vi "TRACEABILITY.vi"() -> ()   [LabVIEW 2017]
uses:
  <vilib>/addons/database/Connection.llb/DB Tools Open Connec (String).vi
  Global/Global 1.vi
  <vilib>/addons/database/NI_Database_API.lvlib
panel:
  in  "Cluster":T1
  out "error out":errorcluster
  in  "error in (no error)":errorcluster
  in  "SAVE":bool
  in  "EXIT":bool
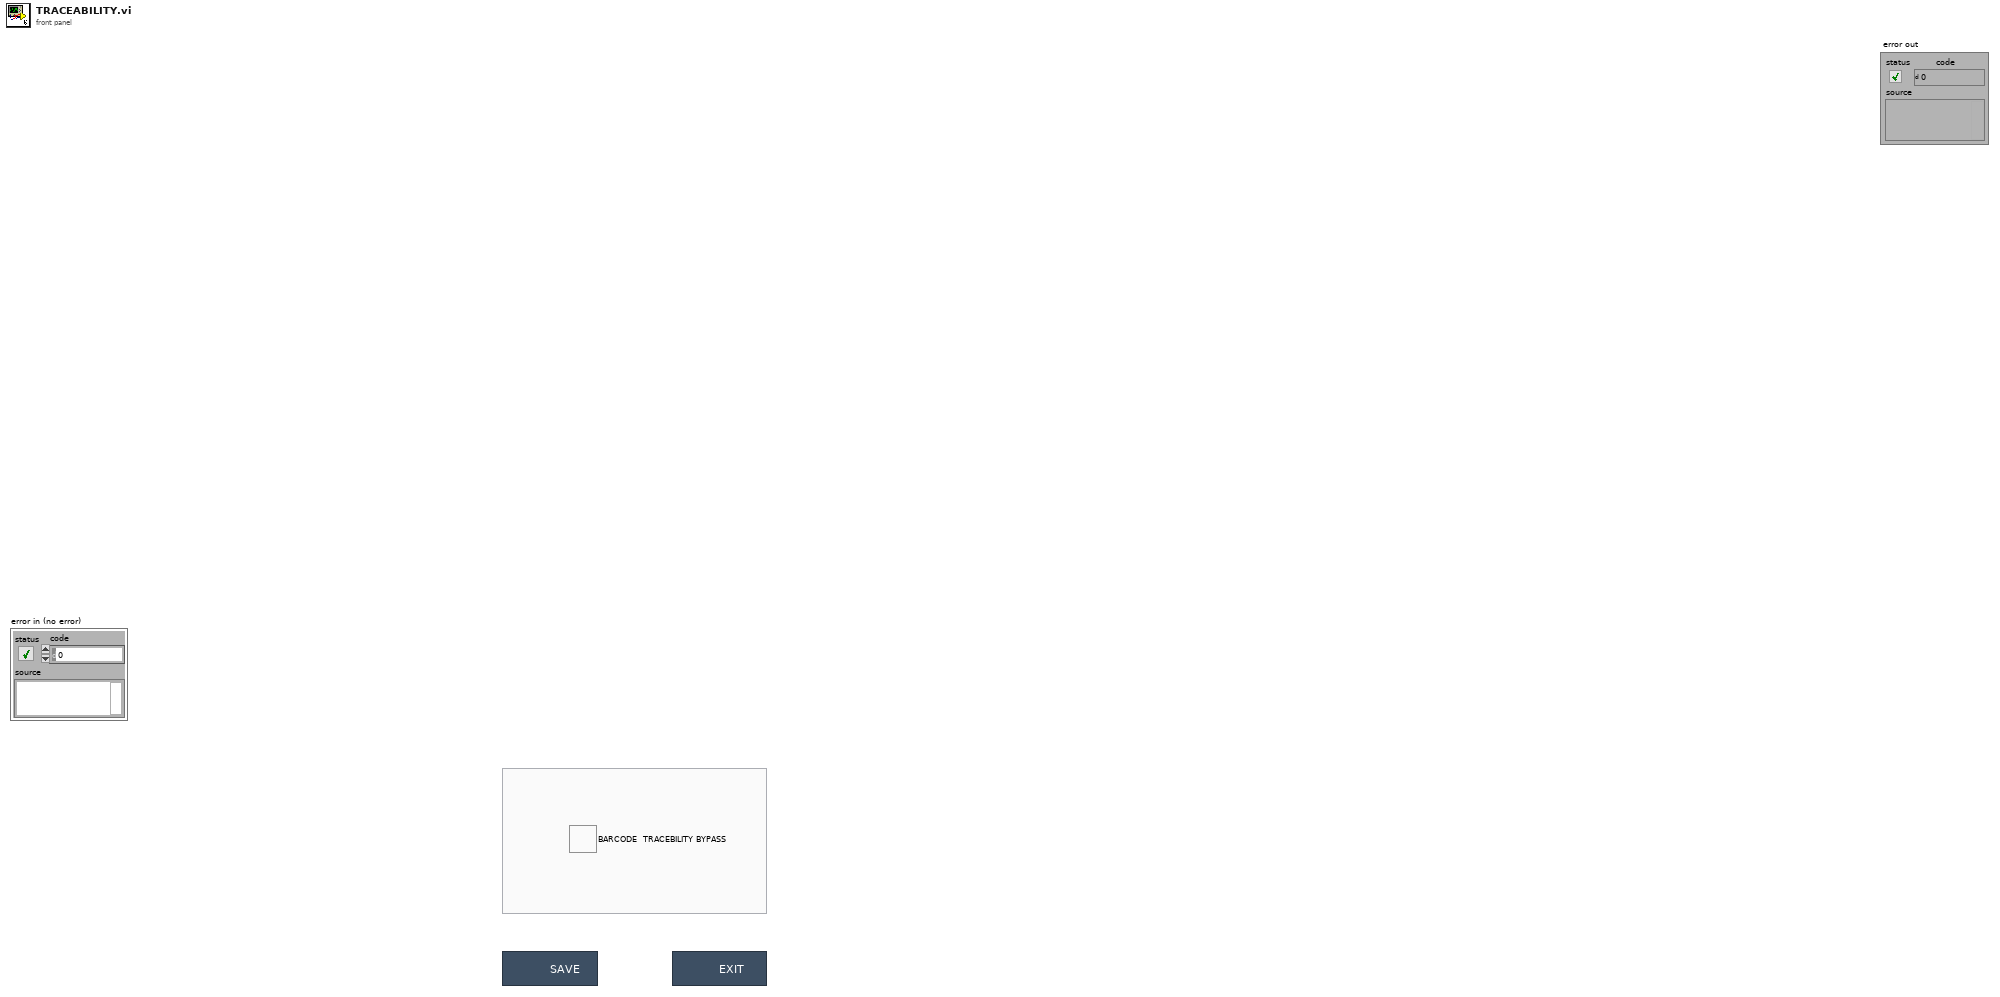
[diagram p1: front panel]
types:
  T1 = cluster{"BARCODE  TRACEBILITY BYPASS":bool, "BOM TRACEABILITY ":bool}
  T2 = cluster{"BARCODE TRACEABILITY":bool, "BOM TRACEABILITY ":bool}
  T3 = typedef "NI_Database_API.lvlib/Conn ObjectReference.ctl" = refnum<k1>
  T4 = enum32{"invalid app kind", "Development System", "Run Time System", "Student Edition", "Embedded LabVIEW", "Evaluation", "Custom"}
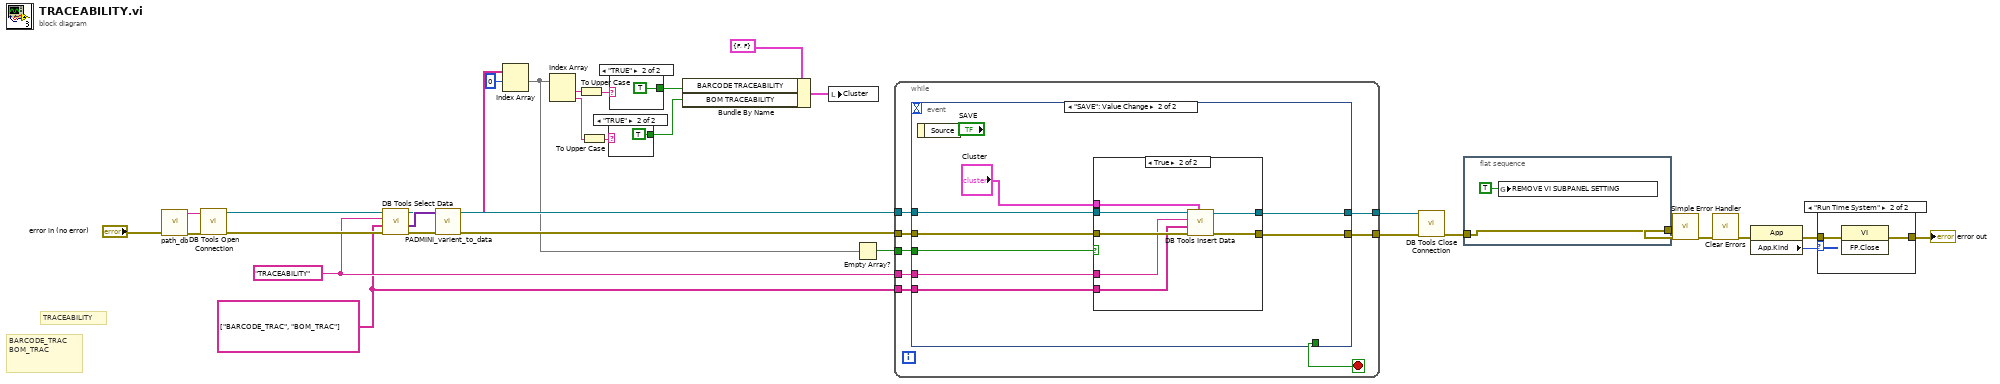
[diagram p0: block diagram]
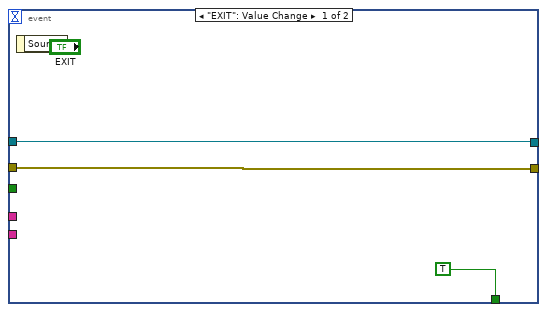
[diagram p2: hidden frame]
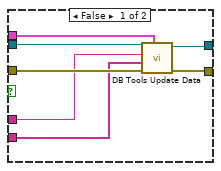
[diagram p3: hidden frame]
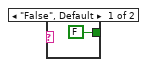
[diagram p5: hidden frame]
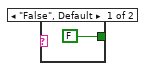
[diagram p6: hidden frame]
diagram:
  w12 = string[] ["BARCODE_TRAC", "BOM_TRAC"] ("columns")
  w13 = "TRACEABILITY" ("table")
  # "BARCODE_TRAC\nBOM_TRAC"
  # "TRACEABILITY"
  n1 = call "path_db.vi"("error in"="error in (no error)") -> ("error out"=w19:errorcluster, "resulting string"=w24:string)  [unwired: 9 in]
  n2 = call-poly <vilib>:"DB Tools Open Connection.vi"("error in (no error)"=w19, "connection information"=w24) -> ("error out"=w23:errorcluster, "connection reference"=w22:T3)  [unwired: 6 in]
  n3 = call <vilib>:"DB Tools Select Data.vi"("error in (no error)"=w23, "columns"=w12, "table"=w13, "connection reference"=w22) -> ("error out"=w21:errorcluster, "data"=w20:variant[][], "connection reference out"=w17:T3)  [unwired: 2 in]
  n4 = call "PADMINI_varient_to_data.vi"("error in (no error)"=w21, "data"=w20) -> ("error out"=w18:errorcluster, "Array"=w15:string[][])  [unwired: 8 in]
  n5 = Index Array(array=w15, index (row)=0 ("disabled index (col)")) -> (element=w14:string[])  [unwired: 1 in]
  n6 = Index Array(array=w14) -> (element #1=w6:string, element #2=w4:string)  [unwired: 2 in]
  n7 = To Upper Case(1:w6) -> (0:w2:string)
  n8 = To Upper Case(1:w4) -> (0:w1:string)
  n9 = case shown="\"TRUE\"" w1 {
    tunnel: [FALSE ("BARCODE TRACEABILITY") TRUE ("BARCODE TRACEABILITY")] -> w3
    frame "False", Default {
    }
    frame "TRUE" {
    }
  }
  n10 = case shown="\"TRUE\"" w2 {
    tunnel: [FALSE ("BARCODE TRACEABILITY") TRUE ("BARCODE TRACEABILITY")] -> w5
    frame "False", Default {
    }
    frame "TRUE" {
    }
  }
  n11 = Bundle By Name(cluster=T2 {"BARCODE TRACEABILITY"=FALSE, "BOM TRACEABILITY "=FALSE} ("Cluster"), "BARCODE TRACEABILITY"=w5, "BOM TRACEABILITY"=w3) -> (w25:T2)
  n12 = local write "Cluster"(w25) -> ()
  n13 = Empty Array?(array=w14) -> (empty?=w16:bool)
  n14 = while {
    tunnel: [w43] -> w10
    tunnel: w18 -> [w44]
    tunnel: w17 -> [w41]
    tunnel: w16 -> [w40]
    tunnel: [w39] -> w11
    tunnel: w13 -> [w38]
    tunnel: w12 -> [w37]
    stop <- w42 stop-if-true
    n15 = event shown="[1] \"SAVE\": Value Change" {
      selector: _ -> [_ _]
      dyn-events: _ -> [_ _]
      timeout: _ -> [_ _]
      tunnel: w44 -> [w47 w54]
      tunnel: [w47 w52] -> w43
      tunnel: [TRUE _] -> w42
      tunnel: w41 -> [w45 w53]
      tunnel: w40 -> [_ w55]
      tunnel: [w45 w51] -> w39
      tunnel: w38 -> [_ w50]
      tunnel: w37 -> [_ w49]
      event "EXIT": Value Change {
        n16 = event-data() -> ()  [unwired: 1 in, 1 out]
      }
      event "SAVE": Value Change {
        n17 = event-data() -> ()  [unwired: 1 in, 1 out]
        n18 = case shown="True" w55 {
          tunnel: w54 -> [w61 w69]
          tunnel: w53 -> [w62 w67]
          tunnel: [w59 w68] -> w52
          tunnel: [w60 w66] -> w51
          tunnel: w50 -> [w58 w65]
          tunnel: w49 -> [w57 w64]
          tunnel: "Cluster" -> [w56 w63]
          frame False {
            n19 = call <vilib>:"DB Tools Update Data.vi"("data"=w56, "error in (no error)"=w61, "columns"=w57, "table"=w58, "connection reference"=w62) -> ("error out"=w59:errorcluster, "connection reference out"=w60:T3)  [unwired: 5 in]
          }
          frame True {
            n20 = call <vilib>:"DB Tools Insert Data.vi"("data"=w63, "error in (no error)"=w69, "columns"=w64, "table"=w65, "connection reference"=w67) -> ("error out"=w68:errorcluster, "connection reference out"=w66:T3)  [unwired: 5 in]
          }
        }
      }
    }
  }
  n21 = call <vilib>:"DB Tools Close Connection.vi"("error in (no error)"=w10, "connection reference"=w11) -> ("error out"=w9:errorcluster)  [unwired: 5 in]
  n22 = flat-sequence {
    tunnel: w9 -> [w71]
    tunnel: [w71] -> w26
    frame #0 {
      n23 = global write "Global 1.vi" "REMOVE VI SUBPANEL SETTING"(TRUE ("REMOVE_VI _SUBPANEL_3")) -> ()
    }
  }
  n24 = call <vilib>:"Simple Error Handler.vi"("error in (no error)"=w26) -> ("error out"=w31:errorcluster)  [unwired: 4 in, 4 out]
  n25 = call <vilib>:"Clear Errors.vi"("error in (no error)"=w31) -> ("error out"=w28:errorcluster)  [unwired: 5 in, 1 out]
  n26 = property class="App"(error in=w28) -> (error out=w29:errorcluster, "App.Kind"=w30:T4)  [unwired: 1 in, 1 out]
  n27 = case shown="\"Run Time System\"" w30 {
    tunnel: w29 -> [w72 w74]
    tunnel: [w72 w73] -> w27
    frame Default {
    }
    frame "Run Time System" {
      n28 = invoke class="VI" method="FP.Close"(error in=w74) -> (error out=w73:errorcluster)  [unwired: 2 in, 2 out]
    }
  }
  "error out" <- w27
